vi "IMIC_Init.vi"(0 "handle":u64=46938896) -> (1 "output param":T1(ring)=enum."failed to open comport", 2 "handle out":u64=46938896)   [LabVIEW 2011]
uses:
  tillimic64.dll
panel:
  out "ips":u8[](array[numeric])
  in  "dummy ips":u8[](array[numeric])
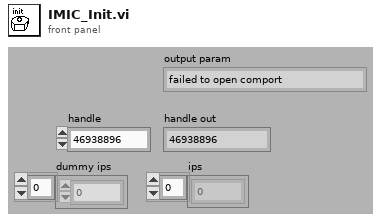
[diagram p1: front panel]
types:
  T1 = enum16{"no error", "missing axis", "missing Z axis", "missing Filter", "iMic not initialized", "no property", "wrong handle", "protocol not finished", "user parameter to long (>32 bits)", "no user parameter handle", "failed to open comport", "failed to initialize"}
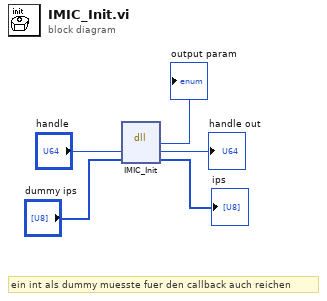
[diagram p0: block diagram]
diagram:
  # "ein int als dummy muesste fuer den callback auch reichen"
  n1 = dll-call lib="C:/Program Files/colibri/Drivers/TILLPhotonics/tillimic*.*" fn="IMIC_Init"("handle"="handle", "ips"="dummy ips") -> ("return type"=→"output param":i32, "handle"=→"handle out":u64, "ips"=→"ips":u8[])  [unwired: 3 in, 2 out]
